vi "close.vi"(8 "error in (no error)":errorcluster, 11 "FgenKeysight in":refnum<class "ArbKeysight.lvclass">) -> (0 "error out":errorcluster)   [LabVIEW 2023, in "ArbKeysight.lvclass"]
doc: "<b>Author:</b> Wolfgang\n<b>Description:</b> This mimics the abilty to close an instrument reference if opened before."
uses:
  ArbKeysight.lvclass
  ArbKeysight.lvclass/ArbKeysight.ctl
  Arb.lvclass
  Driver/Keysight-33500B.lvlib
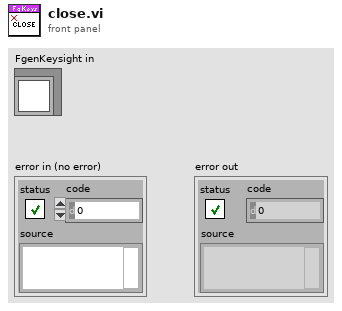
[diagram p1: front panel]
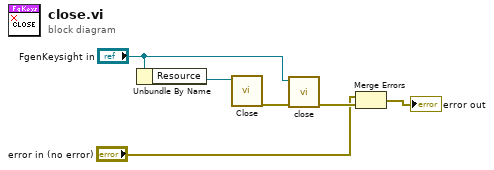
[diagram p0: block diagram]
diagram:
  n1 = Unbundle By Name("FgenKeysight in") -> ("Resource"=w1:refnum<visa-resource-name>)
  n2 = call "Close.vi"("VISA resource name"=w1) -> ("error out"=w5:errorcluster)  [unwired: 10 in]
  n3 = call-parent "close.vi"("error in (no error)"=w5, "Instrument in"="FgenKeysight in") -> ("error out"=w6:errorcluster)  [unwired: 9 in]
  n4 = Merge Errors("error in (no error)", w6) -> (→"error out":errorcluster)
